vi "MFC R clear.vi"(3 "error in":errorcluster) -> (10 "error out":errorcluster)   [LabVIEW 2014]
uses:
  <vilib>/eio/EIOMethodNode/EIOMethodNode.xnode
  <vilib>/rvi/eio/common/nirviEmuTemplateMethod_errors.vi
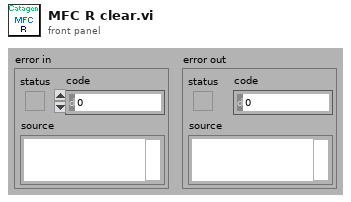
[diagram p1: front panel]
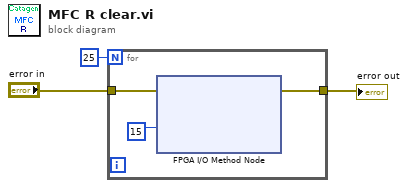
[diagram p0: block diagram]
diagram:
  n1 = for {
    N: 25 -> [_]
    tunnel: "error in" -> [w5]
    tunnel: [w4] -> w1
    n2 = xnode "FPGA I/O Method Node"("error in"=w5, "Timeout (ms)"=15) -> ("error out"=w4:errorcluster)  [unwired: 1 in, 3 out]
  }
  "error out" <- w1
